vi "Temporalcrap.vi"() -> ()   [LabVIEW 2013]
uses:
  <vilib>/Instr/_visa.llb/VISA Configure Serial Port (Instr).vi
panel:
  in  "stop":bool
  in  "up":bool
  in  "downright":bool
  in  "downleft":bool
  in  "upleft":bool
  in  "upright":bool
  in  "right":bool
  in  "left":bool
  in  "down":bool
  in  "BigSmall":bool
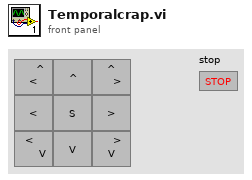
[diagram p1: front panel]
types:
  T1 = cluster{"upleft":bool, "up":bool, "upright":bool, "right":bool, "downright":bool, "down":bool, "downleft":bool, "left":bool, "Bigsmall":bool, "E_stage":errorcluster}
  T2 = cluster{"CH1 AI":tag, "CH1 CI":tag, "CH2 AI":tag, "CH2 CI":tag, "AI X":tag, "AI Y":tag, "AO X-Y":tag, "CH1ST":bool, "CH2ST":bool, "Sigcase":i16, "StageS":i32, "StageL":i32, "data dir":path, "Vp":tag, "Ip":tag, "AO CWlaser":tag, "AO VtoP":tag, "shutter":tag, "488":tag, "532":tag, "640":tag, "LT marker":tag}
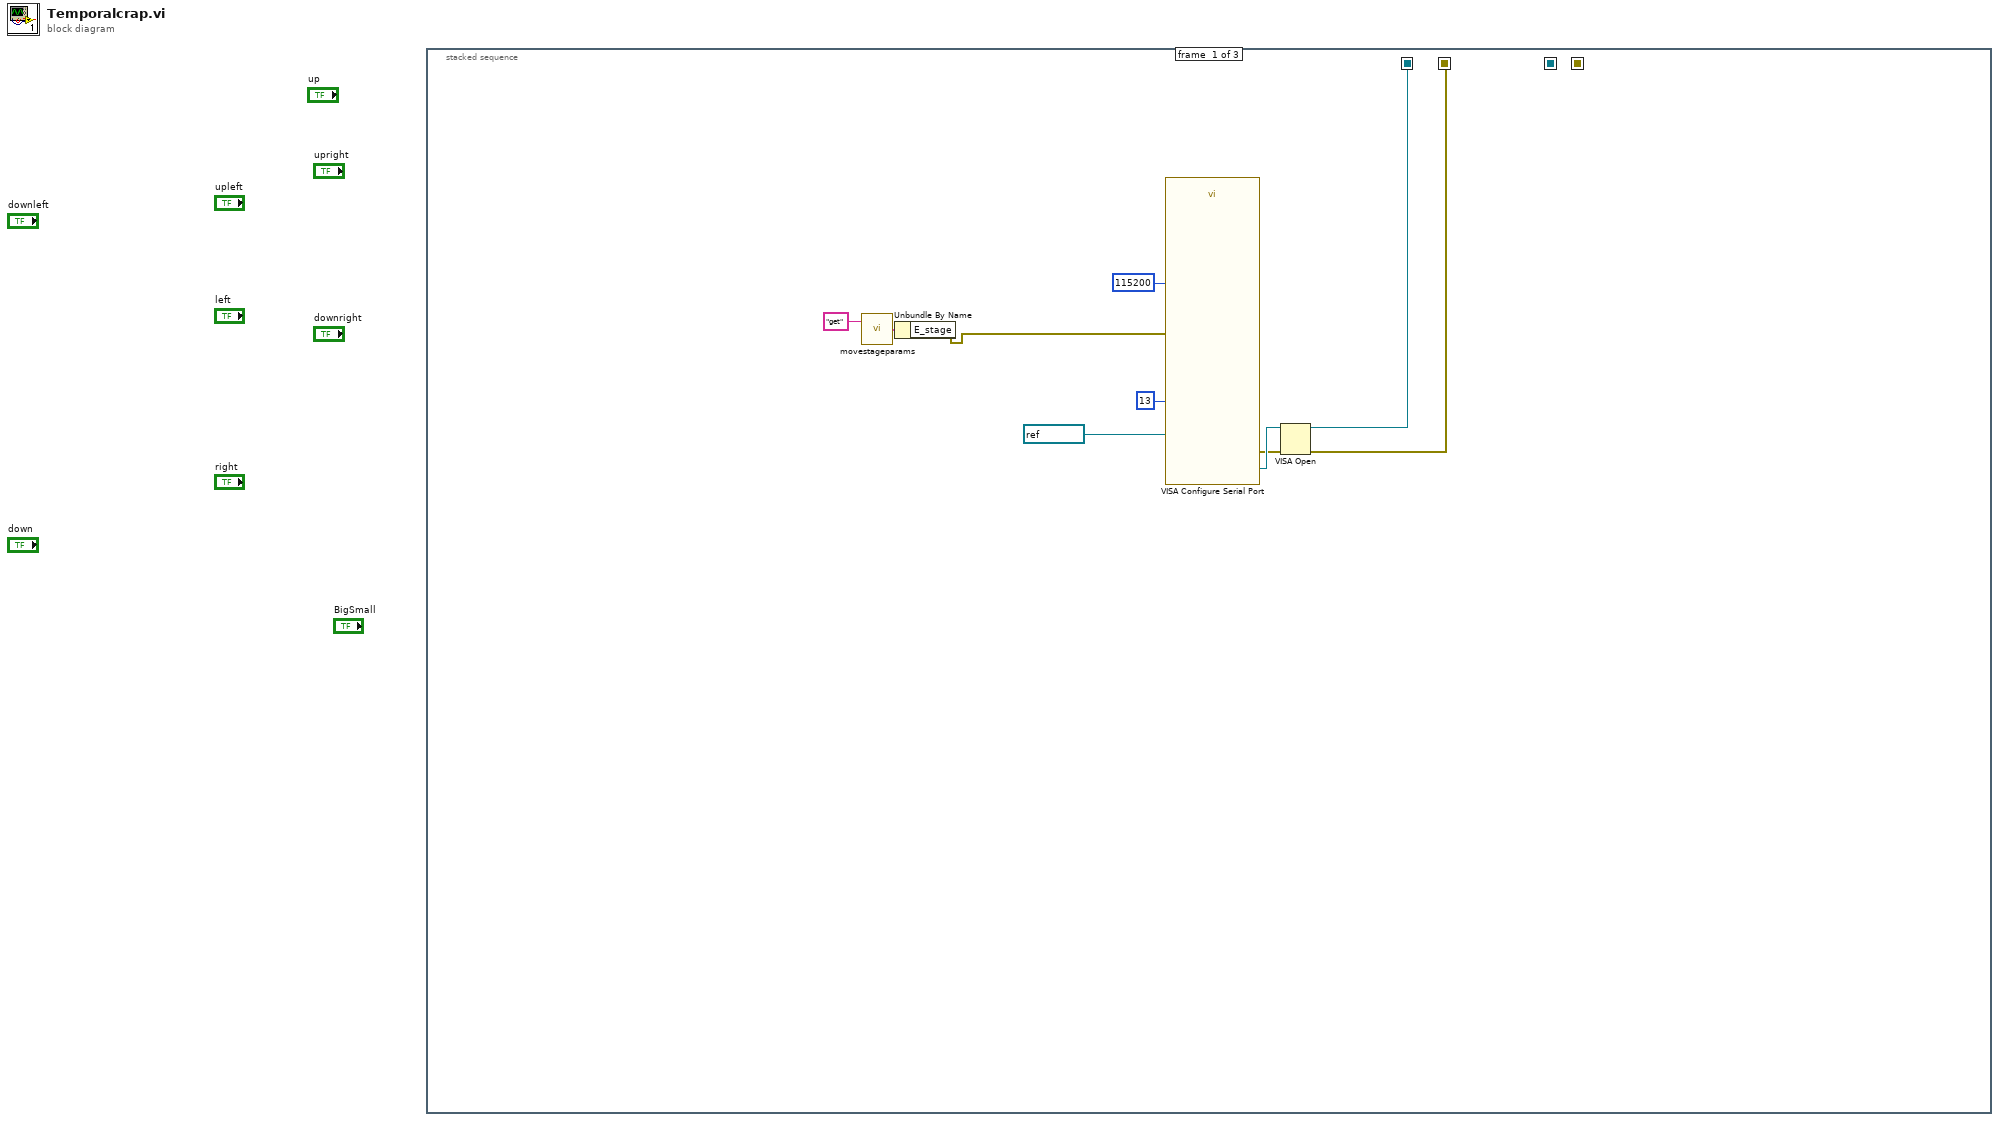
[diagram p0: block diagram]
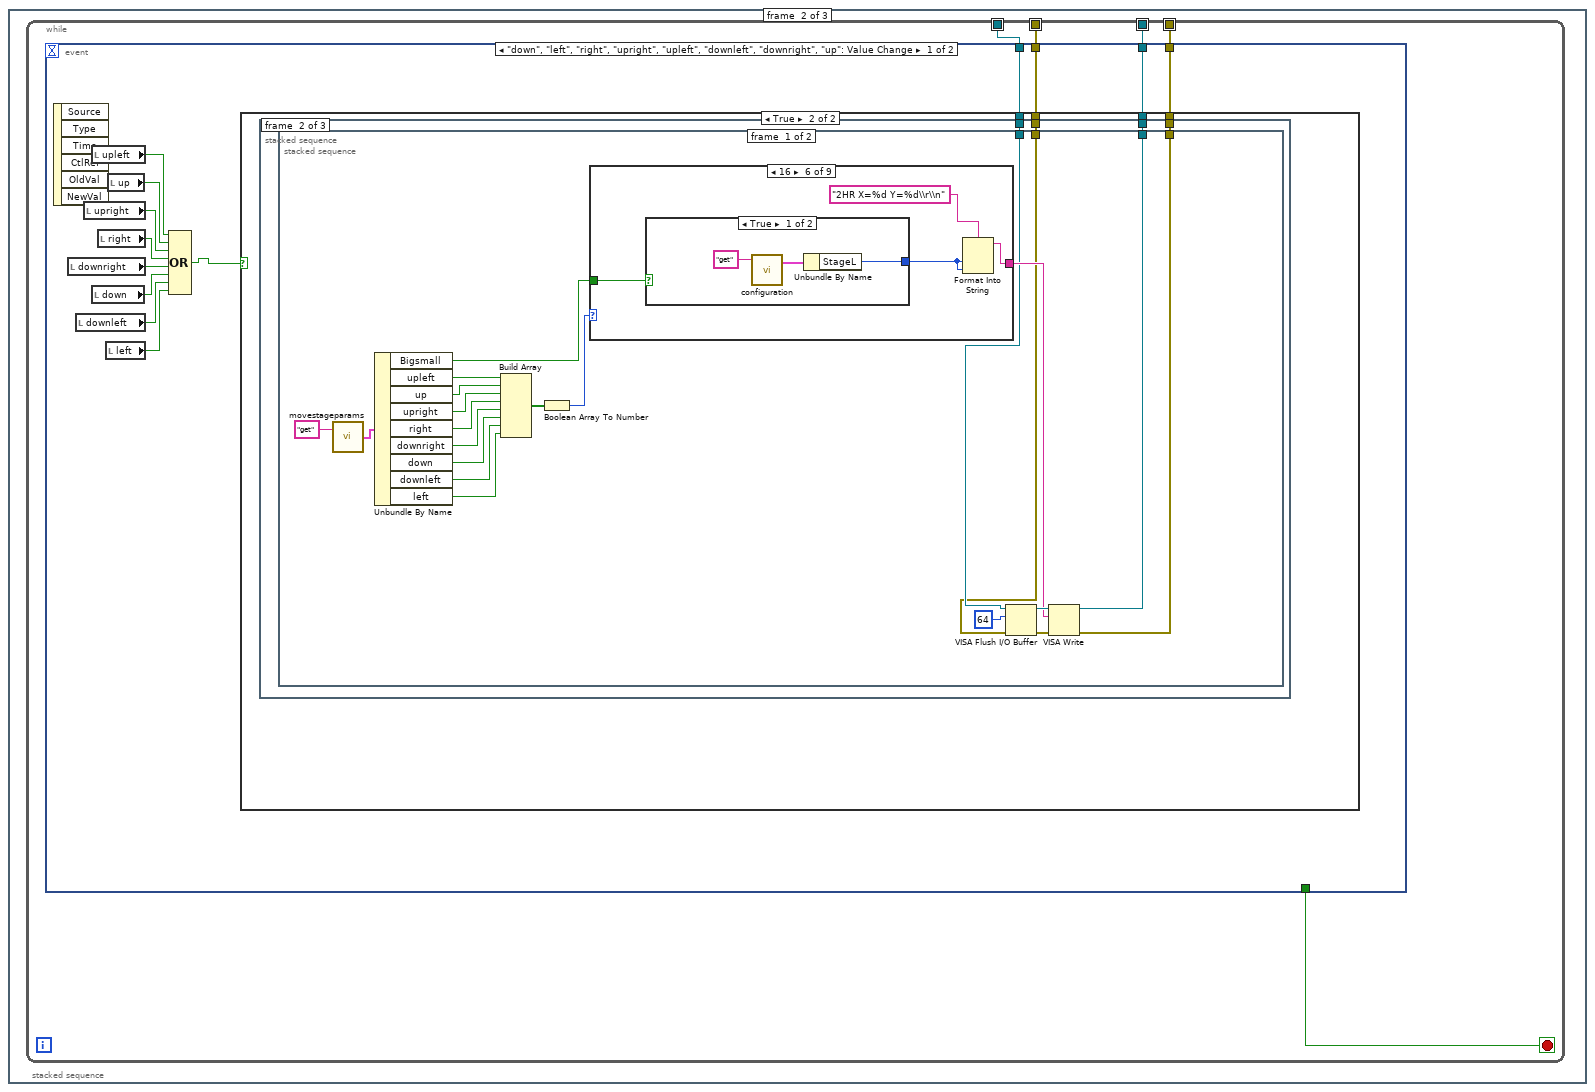
[diagram p2: hidden frame]
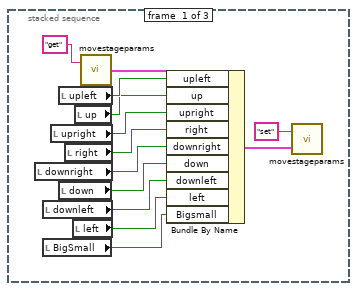
[diagram p4: hidden frame]
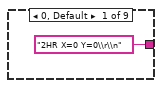
[diagram p5: hidden frame]
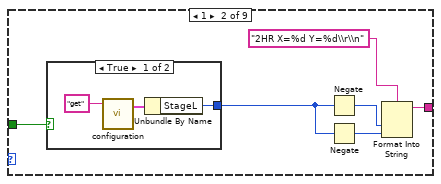
[diagram p6: hidden frame]
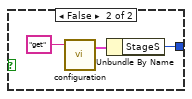
[diagram p7: hidden frame]
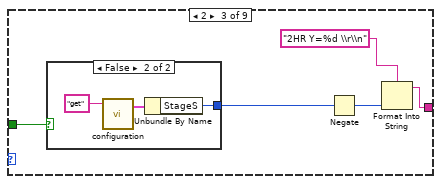
[diagram p8: hidden frame]
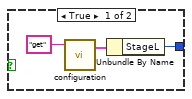
[diagram p9: hidden frame]
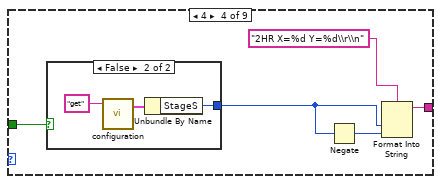
[diagram p10: hidden frame]
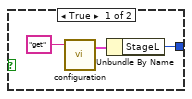
[diagram p11: hidden frame]
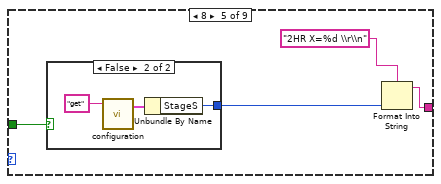
[diagram p12: hidden frame]
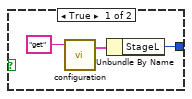
[diagram p13: hidden frame]
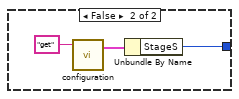
[diagram p14: hidden frame]
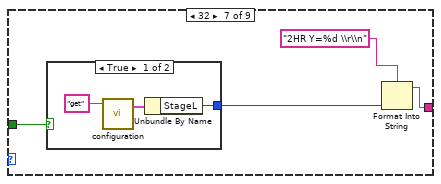
[diagram p15: hidden frame]
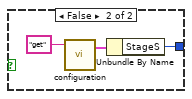
[diagram p16: hidden frame]
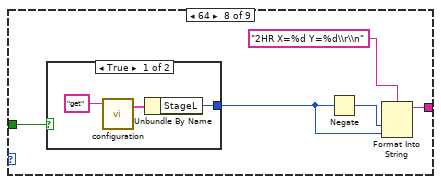
[diagram p17: hidden frame]
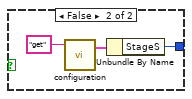
[diagram p18: hidden frame]
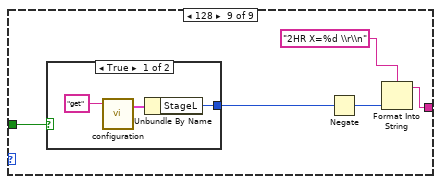
[diagram p19: hidden frame]
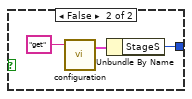
[diagram p20: hidden frame]
diagram:
  n1 = stacked-sequence {
    seq-local: [w2 _ _] -> [_ w14 _]
    seq-local: [w1 _ _] -> [_ w13 _]
    seq-local: [_ w12 _] -> [_ _ w173]
    seq-local: [_ w11 _] -> [_ _ w172]
    frame #0 {
      n2 = call "movestageparams.vi"("command"="get") -> ("Params out"=w4:T1)  [unwired: 1 in]
      n3 = Unbundle By Name(w4) -> ("E_stage"=w3:errorcluster)
      n4 = call-poly "VISA Configure Serial Port"("VISA resource name"=refnum<visa-resource-name> "COM1", "termination char\n(0xA = '\\n' = LF)"=u8 13 ("termination char\n(0xA = '\\n' = LF)"), "baud rate (9600)"=u32 115200 ("baud rate (9600) 2"), "error in (no error)"=w3) -> ("VISA resource name out"=w7:refnum<visa-resource-name>, "error out"=w6:errorcluster)  [unwired: 3 in, 7 out]
      n5 = VISA Open(error in (no error)=w6, VISA resource name=w7) -> (VISA resource name=w2:refnum<visa-resource-name>, error out=w1:errorcluster)  [unwired: 3 in]
    }
    frame #1 {
      n6 = while {
        tunnel: w14 -> [w18]
        tunnel: w13 -> [w17]
        tunnel: [w16] -> w12
        tunnel: [w15] -> w11
        stop <- w19 stop-if-true
        n7 = event shown="[0] \"down\", \"left\", \"right\", \"upright\", \"upleft\", \"downleft\", \"downright\", \"up\": Value Change" {
          selector: _ -> [_ _]
          dyn-events: _ -> [_ _]
          timeout: _ -> [_ _]
          tunnel: [_ "stop"] -> w19
          tunnel: w18 -> [w23 _]
          tunnel: w17 -> [w22 _]
          tunnel: [w21 _] -> w16
          tunnel: [w20 _] -> w15
          event "down", "left", "right", "upright", "upleft", "downleft", "downright", "up": Value Change {
            n8 = event-data() -> ()  [unwired: 1 in, 6 out]
            n9 = local read "downright"() -> (w29:bool)
            n10 = local read "downleft"() -> (w31:bool)
            n11 = local read "upright"() -> (w27:bool)
            n12 = local read "upleft"() -> (w25:bool)
            n13 = local read "down"() -> (w30:bool)
            n14 = local read "right"() -> (w28:bool)
            n15 = local read "left"() -> (w32:bool)
            n16 = local read "up"() -> (w26:bool)
            n17 = Compound Arithmetic op=OR(w25, w26, w27, w28, w29, w30, w31, w32) -> (w24:bool)
            n18 = case shown="True" w24 {
              tunnel: w23 -> [w34 w38]
              tunnel: w22 -> [w33 w37]
              tunnel: [w34 w36] -> w21
              tunnel: [w33 w35] -> w20
              frame False {
              }
              frame True {
                n19 = stacked-sequence {
                  tunnel: w38 -> [_ w55 _]
                  tunnel: w37 -> [_ w54 _]
                  tunnel: [_ w53 _] -> w36
                  tunnel: [_ w52 _] -> w35
                  frame #0 {
                    n20 = local read "downright"() -> (w40:bool)
                    n21 = local read "downleft"() -> (w42:bool)
                    n22 = local read "BigSmall"() -> (w39:bool)
                    n23 = local read "upright"() -> (w44:bool)
                    n24 = local read "upleft"() -> (w47:bool)
                    n25 = local read "down"() -> (w43:bool)
                    n26 = local read "right"() -> (w45:bool)
                    n27 = local read "left"() -> (w41:bool)
                    n28 = local read "up"() -> (w46:bool)
                    n29 = call "movestageparams.vi"("command"="get") -> ("Params out"=w50:T1)  [unwired: 1 in]
                    n30 = Bundle By Name(cluster=w50, "upleft"=w47, "up"=w46, "upright"=w44, "right"=w45, "downright"=w40, "down"=w43, "downleft"=w42, "left"=w41, "Bigsmall"=w39) -> (w51:T1)
                    n31 = call "movestageparams.vi"("Params in"=w51, "command"="set") -> ()  [unwired: 1 out]
                  }
                  frame #1 {
                    n32 = stacked-sequence {
                      tunnel: w55 -> [w59 _]
                      tunnel: w54 -> [w58 _]
                      tunnel: [w57 _] -> w53
                      tunnel: [w56 _] -> w52
                      frame #0 {
                        n33 = call "movestageparams.vi"("command"="get") -> ("Params out"=w67:T1)  [unwired: 1 in]
                        n34 = Unbundle By Name(w67) -> ("Bigsmall"=w76:bool, "upleft"=w68:bool, "up"=w69:bool, "upright"=w70:bool, "right"=w71:bool, "downright"=w72:bool, "down"=w73:bool, "downleft"=w74:bool, "left"=w75:bool)
                        n35 = Build Array(w68, w69, w70, w71, w72, w73, w74, w75) -> (w64:bool[])
                        n36 = Boolean Array To Number(Boolean array=w64) -> (number=w65:u32)
                        n37 = case shown="16" w65 {
                          tunnel: ["2HR X=0 Y=0\\r\\n" w79 w93 w102 w113 w123 w133 w143 w154] -> w60
                          tunnel: w76 -> [_ w78 w90 w101 w112 w122 w132 w142 w153]
                          frame 0, Default {
                          }
                          frame 1 {
                            n38 = case shown="True" w78 {
                              tunnel: [w84 w87] -> w81
                              frame True {
                                n39 = call "configuration.vi"("command"="get") -> ("config out"=w85:T2)  [unwired: 2 in, 1 out]
                                n40 = Unbundle By Name(w85) -> ("StageL"=w84:i32)
                              }
                              frame False {
                                n41 = call "configuration.vi"("command"="get") -> ("config out"=w88:T2)  [unwired: 2 in, 1 out]
                                n42 = Unbundle By Name(w88) -> ("StageS"=w87:i32)
                              }
                            }
                            n43 = Negate(x=w81) -> (-x=w82:i32)
                            n44 = Negate(x=w81) -> (-x=w83:i32)
                            n45 = Format Into String(format string="2HR X=%d Y=%d\\r\\n", w82, w83) -> (resulting string=w79:string)  [unwired: 2 in, 1 out]
                          }
                          frame 2 {
                            n46 = case shown="False" w90 {
                              tunnel: [w95 w98] -> w92
                              frame True {
                                n47 = call "configuration.vi"("command"="get") -> ("config out"=w96:T2)  [unwired: 2 in, 1 out]
                                n48 = Unbundle By Name(w96) -> ("StageL"=w95:i32)
                              }
                              frame False {
                                n49 = call "configuration.vi"("command"="get") -> ("config out"=w99:T2)  [unwired: 2 in, 1 out]
                                n50 = Unbundle By Name(w99) -> ("StageS"=w98:i32)
                              }
                            }
                            n51 = Negate(x=w92) -> (-x=w91:i32)
                            n52 = Format Into String(format string="2HR Y=%d \\r\\n", w91) -> (resulting string=w93:string)  [unwired: 2 in, 1 out]
                          }
                          frame 4 {
                            n53 = case shown="False" w101 {
                              tunnel: [w106 w109] -> w104
                              frame True {
                                n54 = call "configuration.vi"("command"="get") -> ("config out"=w107:T2)  [unwired: 2 in, 1 out]
                                n55 = Unbundle By Name(w107) -> ("StageL"=w106:i32)
                              }
                              frame False {
                                n56 = call "configuration.vi"("command"="get") -> ("config out"=w110:T2)  [unwired: 2 in, 1 out]
                                n57 = Unbundle By Name(w110) -> ("StageS"=w109:i32)
                              }
                            }
                            n58 = Negate(x=w104) -> (-x=w105:i32)
                            n59 = Format Into String(format string="2HR X=%d Y=%d\\r\\n", w104, w105) -> (resulting string=w102:string)  [unwired: 2 in, 1 out]
                          }
                          frame 8 {
                            n60 = case shown="False" w112 {
                              tunnel: [w116 w119] -> w115
                              frame True {
                                n61 = call "configuration.vi"("command"="get") -> ("config out"=w117:T2)  [unwired: 2 in, 1 out]
                                n62 = Unbundle By Name(w117) -> ("StageL"=w116:i32)
                              }
                              frame False {
                                n63 = call "configuration.vi"("command"="get") -> ("config out"=w120:T2)  [unwired: 2 in, 1 out]
                                n64 = Unbundle By Name(w120) -> ("StageS"=w119:i32)
                              }
                            }
                            n65 = Format Into String(format string="2HR X=%d \\r\\n", w115) -> (resulting string=w113:string)  [unwired: 2 in, 1 out]
                          }
                          frame 16 {
                            n66 = case shown="True" w122 {
                              tunnel: [w126 w129] -> w125
                              frame True {
                                n67 = call "configuration.vi"("command"="get") -> ("config out"=w127:T2)  [unwired: 2 in, 1 out]
                                n68 = Unbundle By Name(w127) -> ("StageL"=w126:i32)
                              }
                              frame False {
                                n69 = call "configuration.vi"("command"="get") -> ("config out"=w130:T2)  [unwired: 2 in, 1 out]
                                n70 = Unbundle By Name(w130) -> ("StageS"=w129:i32)
                              }
                            }
                            n71 = Format Into String(format string="2HR X=%d Y=%d\\r\\n", w125, w125) -> (resulting string=w123:string)  [unwired: 2 in, 1 out]
                          }
                          frame 32 {
                            n72 = case shown="True" w132 {
                              tunnel: [w136 w139] -> w134
                              frame True {
                                n73 = call "configuration.vi"("command"="get") -> ("config out"=w137:T2)  [unwired: 2 in, 1 out]
                                n74 = Unbundle By Name(w137) -> ("StageL"=w136:i32)
                              }
                              frame False {
                                n75 = call "configuration.vi"("command"="get") -> ("config out"=w140:T2)  [unwired: 2 in, 1 out]
                                n76 = Unbundle By Name(w140) -> ("StageS"=w139:i32)
                              }
                            }
                            n77 = Format Into String(format string="2HR Y=%d \\r\\n", w134) -> (resulting string=w133:string)  [unwired: 2 in, 1 out]
                          }
                          frame 64 {
                            n78 = case shown="True" w142 {
                              tunnel: [w147 w150] -> w145
                              frame True {
                                n79 = call "configuration.vi"("command"="get") -> ("config out"=w148:T2)  [unwired: 2 in, 1 out]
                                n80 = Unbundle By Name(w148) -> ("StageL"=w147:i32)
                              }
                              frame False {
                                n81 = call "configuration.vi"("command"="get") -> ("config out"=w151:T2)  [unwired: 2 in, 1 out]
                                n82 = Unbundle By Name(w151) -> ("StageS"=w150:i32)
                              }
                            }
                            n83 = Negate(x=w145) -> (-x=w146:i32)
                            n84 = Format Into String(format string="2HR X=%d Y=%d\\r\\n", w146, w145) -> (resulting string=w143:string)  [unwired: 2 in, 1 out]
                          }
                          frame 128 {
                            n85 = case shown="True" w153 {
                              tunnel: [w158 w161] -> w156
                              frame True {
                                n86 = call "configuration.vi"("command"="get") -> ("config out"=w159:T2)  [unwired: 2 in, 1 out]
                                n87 = Unbundle By Name(w159) -> ("StageL"=w158:i32)
                              }
                              frame False {
                                n88 = call "configuration.vi"("command"="get") -> ("config out"=w162:T2)  [unwired: 2 in, 1 out]
                                n89 = Unbundle By Name(w162) -> ("StageS"=w161:i32)
                              }
                            }
                            n90 = Negate(x=w156) -> (-x=w155:i32)
                            n91 = Format Into String(format string="2HR X=%d \\r\\n", w155) -> (resulting string=w154:string)  [unwired: 2 in, 1 out]
                          }
                        }
                        n92 = VISA Flush I/O Buffer(VISA resource name=w59, mask (16)=u16 64, error in (no error)=w58) -> (VISA resource name out=w61:refnum<visa-resource-name>, error out=w62:errorcluster)
                        n93 = VISA Write(VISA resource name=w61, write buffer=w60, error in (no error)=w62) -> (VISA resource name out=w57:refnum<visa-resource-name>, error out=w56:errorcluster)  [unwired: 1 out]
                      }
                      frame #1 {
                        w165 = FALSE
                        n94 = call "movestageparams.vi"("command"="get") -> ("Params out"=w166:T1)  [unwired: 1 in]
                        n95 = Bundle By Name(cluster=w166, "upleft"=w165, "up"=w165, "upright"=w165, "right"=w165, "downright"=w165, "down"=w165, "downleft"=w165, "left"=w165) -> (w164:T1)
                        n96 = call "movestageparams.vi"("Params in"=w164, "command"="set") -> ()  [unwired: 1 out]
                      }
                    }
                  }
                  frame #2 {
                    w169 = FALSE ("OK Button")
                    w170 = FALSE ("OK Button")
                    n97 = property on="down" class="Bool (strict)"("Value"=w170) -> ()  [unwired: 2 in, 2 out]
                    n98 = property on="up" class="Bool (strict)"("Value"=w170) -> ()  [unwired: 2 in, 2 out]
                    n99 = property on="right" class="Bool (strict)"("Value"=w170) -> ()  [unwired: 2 in, 2 out]
                    n100 = property on="left" class="Bool (strict)"("Value"=w170) -> ()  [unwired: 2 in, 2 out]
                    n101 = property on="upright" class="Bool (strict)"("Value"=w169) -> ()  [unwired: 2 in, 2 out]
                    n102 = property on="downleft" class="Bool (strict)"("Value"=w169) -> ()  [unwired: 2 in, 2 out]
                    n103 = property on="downright" class="Bool (strict)"("Value"=w169) -> ()  [unwired: 2 in, 2 out]
                    n104 = property on="upleft" class="Bool (strict)"("Value"=w169) -> ()  [unwired: 2 in, 2 out]
                  }
                }
              }
            }
          }
          event "stop": Value Change {
            n105 = event-data() -> ()  [unwired: 1 in, 6 out]
          }
        }
      }
    }
    frame #2 {
      n106 = call "movestageparams.vi"("command"="get") -> ("Params out"=w176:T1)  [unwired: 1 in]
      n107 = VISA Close(VISA resource name=w173, error in (no error)=w172) -> (error out=w177:errorcluster)
      n108 = Bundle By Name(cluster=w176, "E_stage"=w177) -> (w178:T1)
      n109 = call "movestageparams.vi"("Params in"=w178, "command"="set") -> ()  [unwired: 1 out]
    }
  }
